vi "Viewer.vi"() -> ()   [LabVIEW 2009]
uses:
  <vilib>/Platform/TimedLoop/XDataNode/XDataNode.xnode
  <vilib>/Platform/TimedLoop/XDataNode/loadlvalarms.vi
  <vilib>/Platform/TimedLoop/XDataNode/timing_clust.ctl
  <vilib>/Platform/TimedLoop/XDataNode/nitl_modes.ctl
  <vilib>/Platform/TimedLoop/XDataNode/wakeup.ctl
  UDP Lib/UDP Network Location.ctl
  <vilib>/Platform/TimedLoop/XDataNode/XDNodeRunTimeDep.lvlib
panel:
  out "Count out":i32
  in  "stop":bool
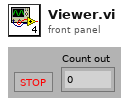
[diagram p1: front panel]
types:
  T1 = typedef "UDP Base.ctl" = cluster{"UDP Session":refnum<k16>, "UDP Socket Params":T2}
  T2 = typedef "UDP Socket Params.ctl" = cluster{"Local Port":u16, "Read Timeout":i32, "Write Timeout":i32}
  T3 = typedef "XDNodeRunTimeDep.lvlib/timing_clust.ctl" = cluster{"Expected End [f-1]":u64, "Actual End [f-1]":u64, "Finished Late? [f-1]":bool, "Expected End [i-1]":u64, "Actual End [i-1]":u64, "Finished Late? [i-1]":bool, "Expected Start [i]":u64, "Actual Start [i]":u64, "Expected Start [f]":u64, "Actual Start [f]":u64, "Source Name":string, "Structure Name":string, "Period":i64, "Deadline":i64, "Offset":i64, "Start":i64, "Priority":i32, "Timeout":i32, "Mode":T4, "Wakeup Reason":T5, "Error":errorcluster, "Source Type":string, "Secondary Source Type":string, "Global End Time":u64, "Global Start Time":u64, "Frame Duration":u64, "Iteration Duration":u64, "Assigned CPU":i32, "I/O Scan Engine Mode":u32}
  T4 = typedef "XDNodeRunTimeDep.lvlib/nitl_modes.ctl" = enum32{"No Change", "Process missed periods, maintain original phase", "Discard missed periods, maintain original phase", "Process missed periods, ignore original phase", "Discard missed periods, ignore original phase"}
  T5 = typedef "XDNodeRunTimeDep.lvlib/wakeup.ctl" = enum32{"Normal", "Aborted", "Asynchronous wakeup", "Timing source error", "Timed loop error", "Timeout"}
  T6 = typedef "UDP Network Location.ctl" = cluster{"IP Address":string, "Port":u16}
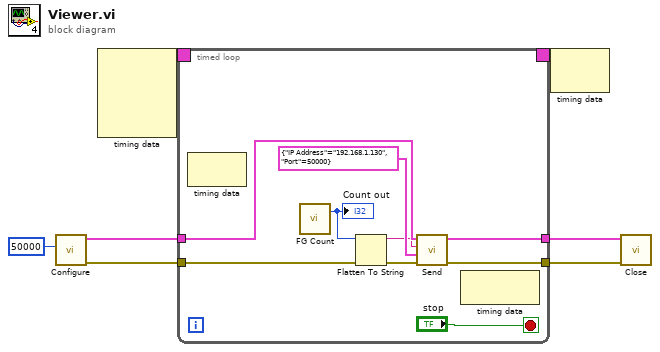
[diagram p0: block diagram]
diagram:
  n1 = call "Configure.vi"("Local Port"=u16 50000) -> ("error out"=w5:errorcluster, "UDP Base out"=w4:T1)  [unwired: 9 in]
  n2 = node-c288() -> (w7:T3)  [unwired: 4 in]
  n3 = timed-loop {
    timing: w7 -> [_]
    timing-out: [_] -> w6
    tunnel: w5 -> [w9]
    tunnel: w4 -> [w14]
    tunnel: [w13] -> w2
    tunnel: [w12] -> w1
    stop <- "stop" stop-if-true
    n4 = node-c288() -> ()  [unwired: 1 in, 1 out]
    n5 = call "FG Count.vi"() -> ("Count out"=w11:i32)  [unwired: 3 in]
    "Count out" <- w11
    n6 = Flatten To String(anything=w11, error in (no error)=w9) -> (data string=w10:string, error out=w8:errorcluster)  [unwired: 2 in, 1 out]
    n7 = call "Send.vi"("error in (no error)"=w8, "Destination Location"=T6 {"IP Address"="192.168.1.130", "Port"=50000}, "Send Data"=w10, "UDP Base in"=w14) -> ("error out"=w12:errorcluster, "UDP Base out"=w13:T1)  [unwired: 5 in, 1 out]
    n8 = node-c288() -> ()  [unwired: 1 in, 1 out]
  }
  n9 = node-c288(w6) -> ()  [unwired: 1 out]
  n10 = call "Close.vi"("error in (no error)"=w1, "Cluster of class private data"=w2) -> ()  [unwired: 9 in, 1 out]
